vi "test - Cluster mixed with Array.vi"(8 "error in (no error)":errorcluster, 11 "TestCase in":refnum<class "testcase-Supported-Datatype.lvclass">) -> (0 "error out":errorcluster, 3 "TestCase out":refnum<class "testcase-Supported-Datatype.lvclass">)   [LabVIEW 2017, in "testcase-Supported-Datatype.lvclass"]
uses:
  testcase-Supported-Datatype.lvclass
  bf0868fe-d351-4dd5-b7ea-1ae6d7303ec2.vi
  bc29c70e-f259-45b6-837b-c6db9792f216.vi
  21070344-a214-4798-b894-728e681e4f24.vi
  a587c1a0-4a74-4f4f-b260-525f07160d7a.vi
  523d1283-6dc0-47eb-92bf-acf823cb1d85.vi
  47cfac6e-2fb6-42ac-b8f8-2f4224af837d.vi
  addons/API-String-Arugments-Support/_Support/Data To API String Arguments.vi
  <vilib>/addons/_JKI Toolkits/VI Tester/TestCase.llb/TestCase.lvclass
  addons/API-String-Arugments-Support/API String Arguments Support.lvlib
  C:/Program Files (x86)/National Instruments/LabVIEW 2017/vi.lib/addons/_JKI Toolkits/VI Tester/TestCase.llb/TestCase.lvclass
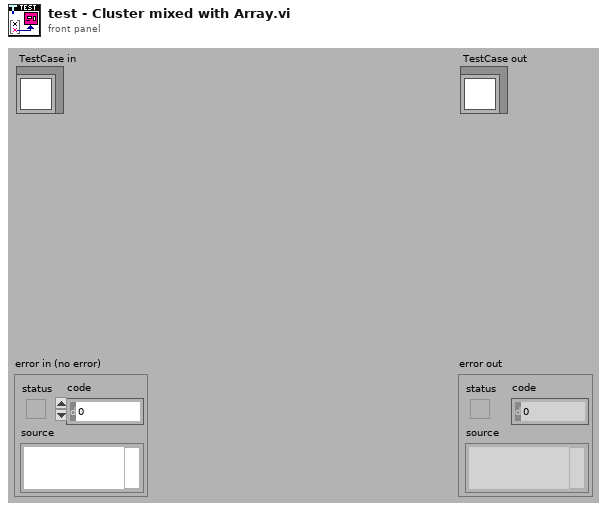
[diagram p1: front panel]
types:
  T1 = cluster{"String":string, "Numberic":i32, "Boolean":bool, "1D Array":dbl[], "2D Array":dbl[][], "Cluster":cluster{"String":string, "Numberic":i32, "Boolean":bool, "1D Array":dbl[], "2D Array":dbl[][]}}
  T2 = cluster{"String":string, "Numberic":i32, "Boolean":bool, "1D Array":dbl[], "2D Array":dbl[][]}
  T3 = cluster{"String":string, "Numberic":i32, "Boolean":bool, "1D Array":dbl[], "2D Array":dbl[][], "Cluster":cluster{"String":string, "Numberic":i32, "Boolean":bool}}[]
  T4 = cluster{"String":string, "Numberic":i32, "Boolean":bool, "1D Array":dbl[], "2D Array":dbl[][], "Cluster":cluster{"String":string, "Numberic":i32, "Boolean":bool, "1D Array":dbl[], "2D Array":dbl[][]}}[]
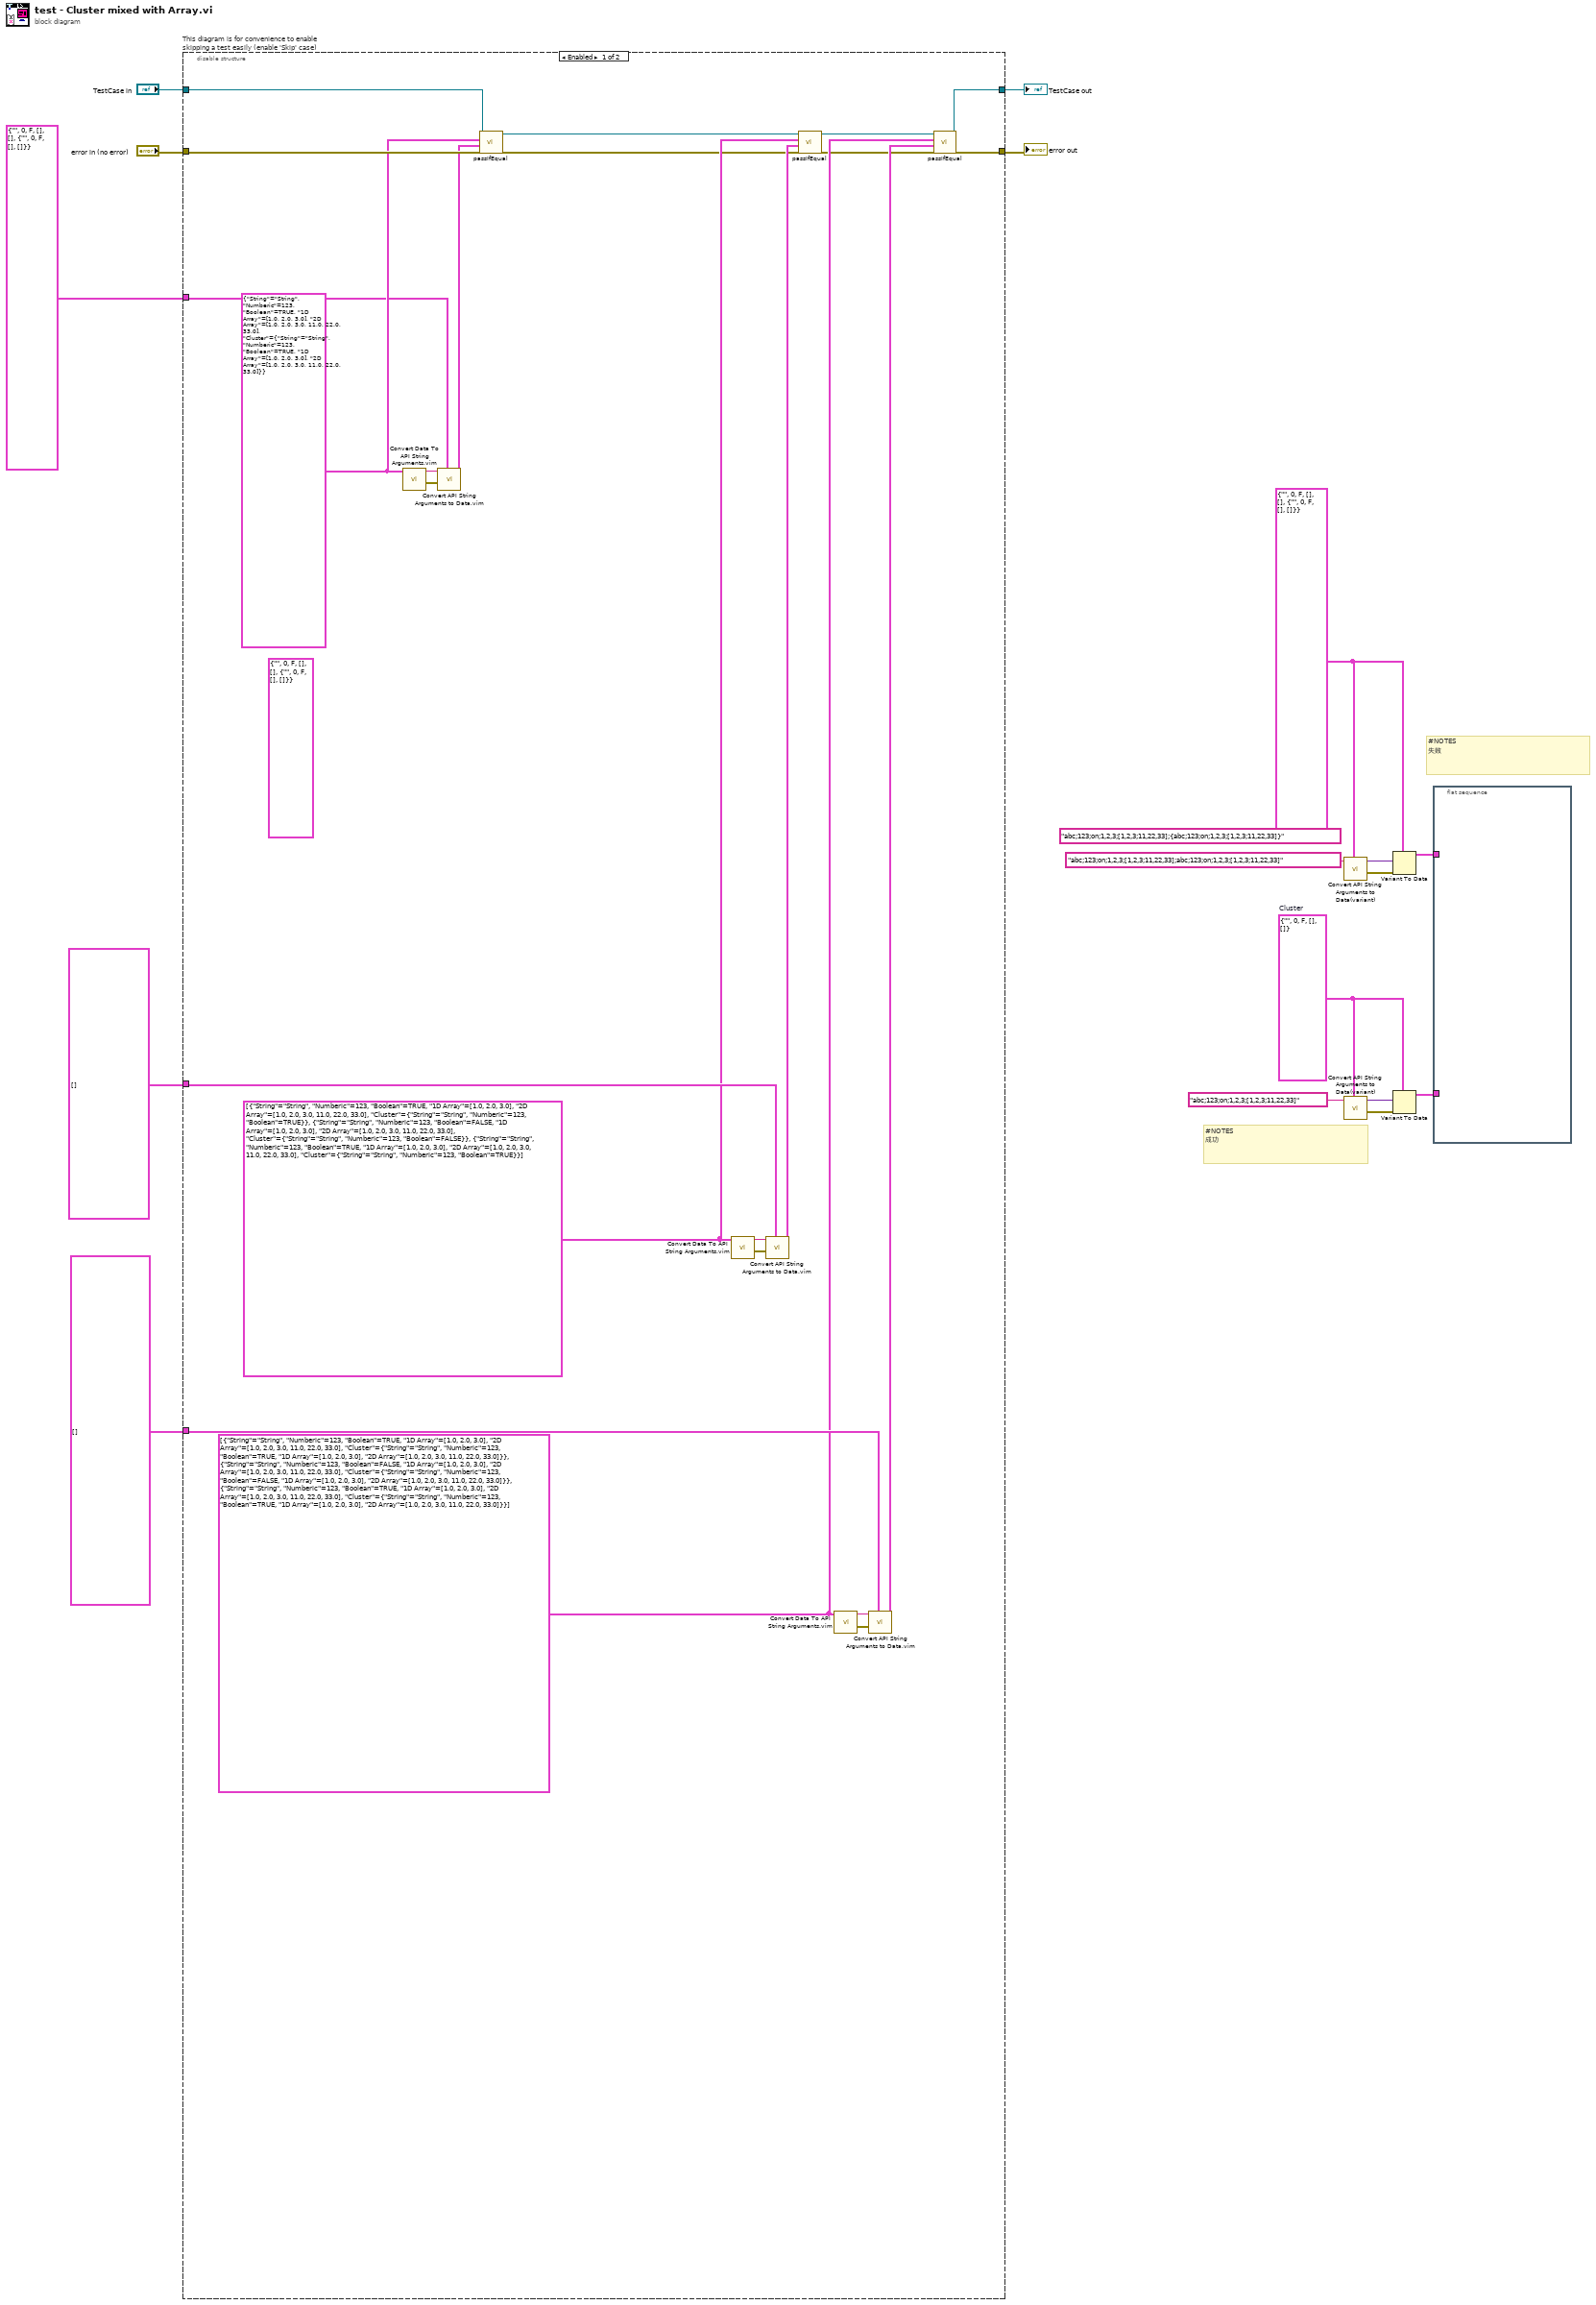
[diagram p0: block diagram]
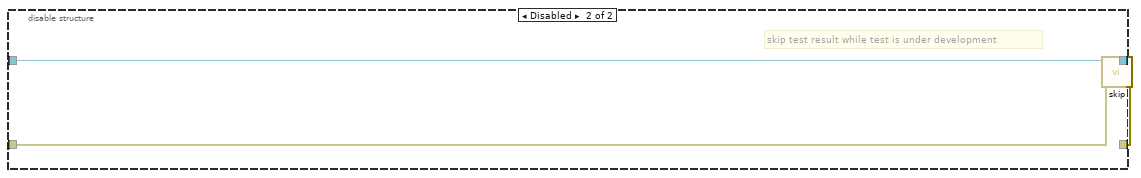
[diagram p2: hidden frame]
diagram:
  (unwired) "abc;123;on;1,2,3;[1,2,3;11,22,33];{abc;123;on;1,2,3;[1,2,3;11,22,33]}" ("String")
  w4 = T1 {"String"="", "Numberic"=0, "Boolean"=FALSE, "1D Array"=[], "2D Array"=[], "Cluster"={"String"="", "Numberic"=0, "Boolean"=FALSE, "1D Array"=[], "2D Array"=[]}}
  w7 = T2 {"String"="", "Numberic"=0, "Boolean"=FALSE, "1D Array"=[], "2D Array"=[]}  # Cluster
  # "#NOTES\n成功"
  # "#NOTES\n失败"
  n1 = disable-structure "This diagram is for convenience to enable skipping a test easily (enable 'Skip' case)" shown="Enabled" {
    disable-tunnel: "TestCase in" -> [w40 w44]
    disable-tunnel: [w37 w42] -> w14
    disable-tunnel: [w38 w43] -> w16
    disable-tunnel: "error in (no error)" -> [w39 w41]
    disable-tunnel: T4 [] -> [w30 _]
    disable-tunnel: T1 {"String"="", "Numberic"=0, "Boolean"=FALSE, "1D Array"=[], "2D Array"=[], "Cluster"={"String"="", "Numberic"=0, "Boolean"=FALSE, "1D Array"=[], "2D Array"=[]}} -> [w29 _]
    disable-tunnel: T3 [] -> [w24 _]
    frame Enabled {
      (unwired) T1 {"String"="", "Numberic"=0, "Boolean"=FALSE, "1D Array"=[], "2D Array"=[], "Cluster"={"String"="", "Numberic"=0, "Boolean"=FALSE, "1D Array"=[], "2D Array"=[]}} ("Data")
      w21 = T3 [{"String"="String", "Numberic"=123, "Boolean"=TRUE, "1D Array"=[1.0, 2.0, 3.0], "2D Array"=[[1.0, 2.0, 3.0], [11.0, 22.0, 33.0]], "Cluster"={"String"="String", "Numberic"=123, "Boolean"=TRUE}}, {"String"="String", "Numberic"=123, "Boolean"=FALSE, "1D Array"=[1.0, 2.0, 3.0], "2D Array"=[[1.0, 2.0, 3.0], [11.0, 22.0, 33.0]], "Cluster"={"String"="String", "Numberic"=123, "Boolean"=FALSE}}, {"String"="String", "Numberic"=123, "Boolean"=TRUE, "1D Array"=[1.0, 2.0, 3.0], "2D Array"=[[1.0, 2.0, 3.0], [11.0, 22.0, 33.0]], "Cluster"={"String"="String", "Numberic"=123, "Boolean"=TRUE}}]
      w27 = T4 [{"String"="String", "Numberic"=123, "Boolean"=TRUE, "1D Array"=[1.0, 2.0, 3.0], "2D Array"=[[1.0, 2.0, 3.0], [11.0, 22.0, 33.0]], "Cluster"={"String"="String", "Numberic"=123, "Boolean"=TRUE, "1D Array"=[1.0, 2.0, 3.0], "2D Array"=[[1.0, 2.0, 3.0], [11.0, 22.0, 33.0]]}}, {"String"="String", "Numberic"=123, "Boolean"=FALSE, "1D Array"=[1.0, 2.0, 3.0], "2D Array"=[[1.0, 2.0, 3.0], [11.0, 22.0, 33.0]], "Cluster"={"String"="String", "Numberic"=123, "Boolean"=FALSE, "1D Array"=[1.0, 2.0, 3.0], "2D Array"=[[1.0, 2.0, 3.0], [11.0, 22.0, 33.0]]}}, {"String"="String", "Numberic"=123, "Boolean"=TRUE, "1D Array"=[1.0, 2.0, 3.0], "2D Array"=[[1.0, 2.0, 3.0], [11.0, 22.0, 33.0]], "Cluster"={"String"="String", "Numberic"=123, "Boolean"=TRUE, "1D Array"=[1.0, 2.0, 3.0], "2D Array"=[[1.0, 2.0, 3.0], [11.0, 22.0, 33.0]]}}]
      w34 = T1 {"String"="String", "Numberic"=123, "Boolean"=TRUE, "1D Array"=[1.0, 2.0, 3.0], "2D Array"=[[1.0, 2.0, 3.0], [11.0, 22.0, 33.0]], "Cluster"={"String"="String", "Numberic"=123, "Boolean"=TRUE, "1D Array"=[1.0, 2.0, 3.0], "2D Array"=[[1.0, 2.0, 3.0], [11.0, 22.0, 33.0]]}}
      n2 = call "Convert Data To API String Arguments.vim"("Data"=w34) -> ("error out"=w36:errorcluster, "API String"=w35:string)  [unwired: 7 in]
      n3 = call "Convert API String Arguments to Data.vim"("Reference Type"=w29, "error in (no error)"=w36, "API String"=w35) -> ("Data"=w33:T1)  [unwired: 5 in, 1 out]
      n4 = call-dynamic "passIfEqual.vi"("error in (no error)"=w39, "y"=w33, "x"=w34, "TestCase in"=w40) -> ("error out"=w18:errorcluster, "TestCase out"=w19:refnum<class "testcase-Supported-Datatype.lvclass">)  [unwired: 6 in]
      n5 = call "Convert Data To API String Arguments.vim"("Data"=w21) -> ("error out"=w26:errorcluster, "API String"=w25:string)  [unwired: 7 in]
      n6 = call "Convert API String Arguments to Data.vim"("Reference Type"=w24, "error in (no error)"=w26, "API String"=w25) -> ("Data"=w20:T3)  [unwired: 5 in, 1 out]
      n7 = call-dynamic "passIfEqual.vi"("error in (no error)"=w18, "y"=w20, "x"=w21, "TestCase in"=w19) -> ("error out"=w22:errorcluster, "TestCase out"=w23:refnum<class "testcase-Supported-Datatype.lvclass">)  [unwired: 6 in]
      n8 = call "Convert Data To API String Arguments.vim"("Data"=w27) -> ("error out"=w31:errorcluster, "API String"=w32:string)  [unwired: 7 in]
      n9 = call "Convert API String Arguments to Data.vim"("Reference Type"=w30, "error in (no error)"=w31, "API String"=w32) -> ("Data"=w28:T4)  [unwired: 5 in, 1 out]
      n10 = call-dynamic "passIfEqual.vi"("error in (no error)"=w22, "y"=w28, "x"=w27, "TestCase in"=w23) -> ("error out"=w38:errorcluster, "TestCase out"=w37:refnum<class "testcase-Supported-Datatype.lvclass">)  [unwired: 6 in]
    }
    frame Disabled {
      # "skip test result while test is under development"
      n11 = call <vilib>:"skip.vi"("error in (no error)"=w41, "TestCase in"=w44) -> ("error out"=w43:errorcluster, "TestCase out"=w42:refnum<class "testcase-Supported-Datatype.lvclass">)  [unwired: 8 in]
    }
  }
  "error out" <- w16
  "TestCase out" <- w14
  n12 = call "Convert API String Arguments to Data(variant).vi"("Type"=w4, "String"="abc;123;on;1,2,3;[1,2,3;11,22,33];abc;123;on;1,2,3;[1,2,3;11,22,33]") -> ("error"=w6:errorcluster, "Data"=w5:variant)  [unwired: 8 in]
  n13 = call "Convert API String Arguments to Data(variant).vi"("Type"=w7, "String"="abc;123;on;1,2,3;[1,2,3;11,22,33]") -> ("error"=w9:errorcluster, "Data"=w10:variant)  [unwired: 8 in]
  n14 = Variant To Data(error in=w6, type=w4, Variant=w5) -> (data=w2:T1)  [unwired: 1 out]
  n15 = Variant To Data(error in=w9, type=w7, Variant=w10) -> (data=w1:T2)  [unwired: 1 out]
  n16 = flat-sequence {
    tunnel: w2 -> [_]
    tunnel: w1 -> [_]
    frame #0 {
    }
  }
